vi "Data_get_joe_1.vi"() -> ()   [LabVIEW 2011]
uses:
  <vilib>/Analysis/2dsp.llb/Real FFT.vi
  <vilib>/Analysis/NI_AALPro.lvlib
panel:
  in  "Automatic Overwrite?":bool
  out "f cur. (GHz)":i32
  in  "TDS VISA Port":refnum<visa-resource-name>="GPIB0::1::INSTR"
  in  "Chirp up to (GHz)":dbl
  in  "PauseB":bool caption="Pause"
  in  "Substr":bool
  out "tdsavges#":i32 caption="tds averaged:"
  in  "Auto":bool caption="Autosave"
  in  "FFT every#":u32=1 min=1 max=1000 step=1
  in  "#steps":u32=1 min=1 step=1
  in  "f step (MHz)":dbl=0.0003 min=0.00025 max=67.0 step=1e-06 format="%#.12f"
  in  "time/point":T1(ring)
  in  "time/div":T2(ring)
  out "Current sweep":u32=1 min=1 max=1000 step=1
  in  "Ext":string="ccd"
  in  "Name":string="trace"
  in  "Folder":path
  in  "#Sweeps":u32=1 min=1 max=1000 step=1
  in  "Ampl. (dBm)":dbl min=-135.0 max=30.0 step=0.5 format="%#_8g"
  in  "f start (GHz)":dbl=0.0003 min=0.00025 max=67.0 step=1e-06 format="%#.12f"
  in  "Start":bool
  in  "Quit":bool
  in  "E8257D VISA Port":refnum<visa-resource-name>="GPIB0::1::INSTR"
  out "read time (ms)":u32
  out "#points":u32
  out "Busy":bool
  in  "Repetition rate (Hz)":ext=2.5
  in  "Chirp start (MHz)":ext=2.5
  in  "Filter up to (MHz)":ext=2.5
  in  "Amount of averagings":u32=10 min=1 step=1
  out "Data":dbl[](array[numeric])
  out "Frequency Domain Signal":cluster{ext[], dbl[]}(graph)
  out "FFT (Im)":dbl[](array[numeric])
  out "FFT (Re)":dbl[](array[numeric])
  out "Final array":ext[][](array[numeric])
  out "size(s)":i32
  out "Oscilloscope Data":dbl[](array[numeric])
  in  "Channel Number":u16=1
  out "Oscilloscope graph":dbl[](graph)
  in  "Stop":bool
  # "Oscilloscope TDS6124C"
  # "File Storage"
  # "PSG E8257D"
  # "Control"
  # "Spectrum data"
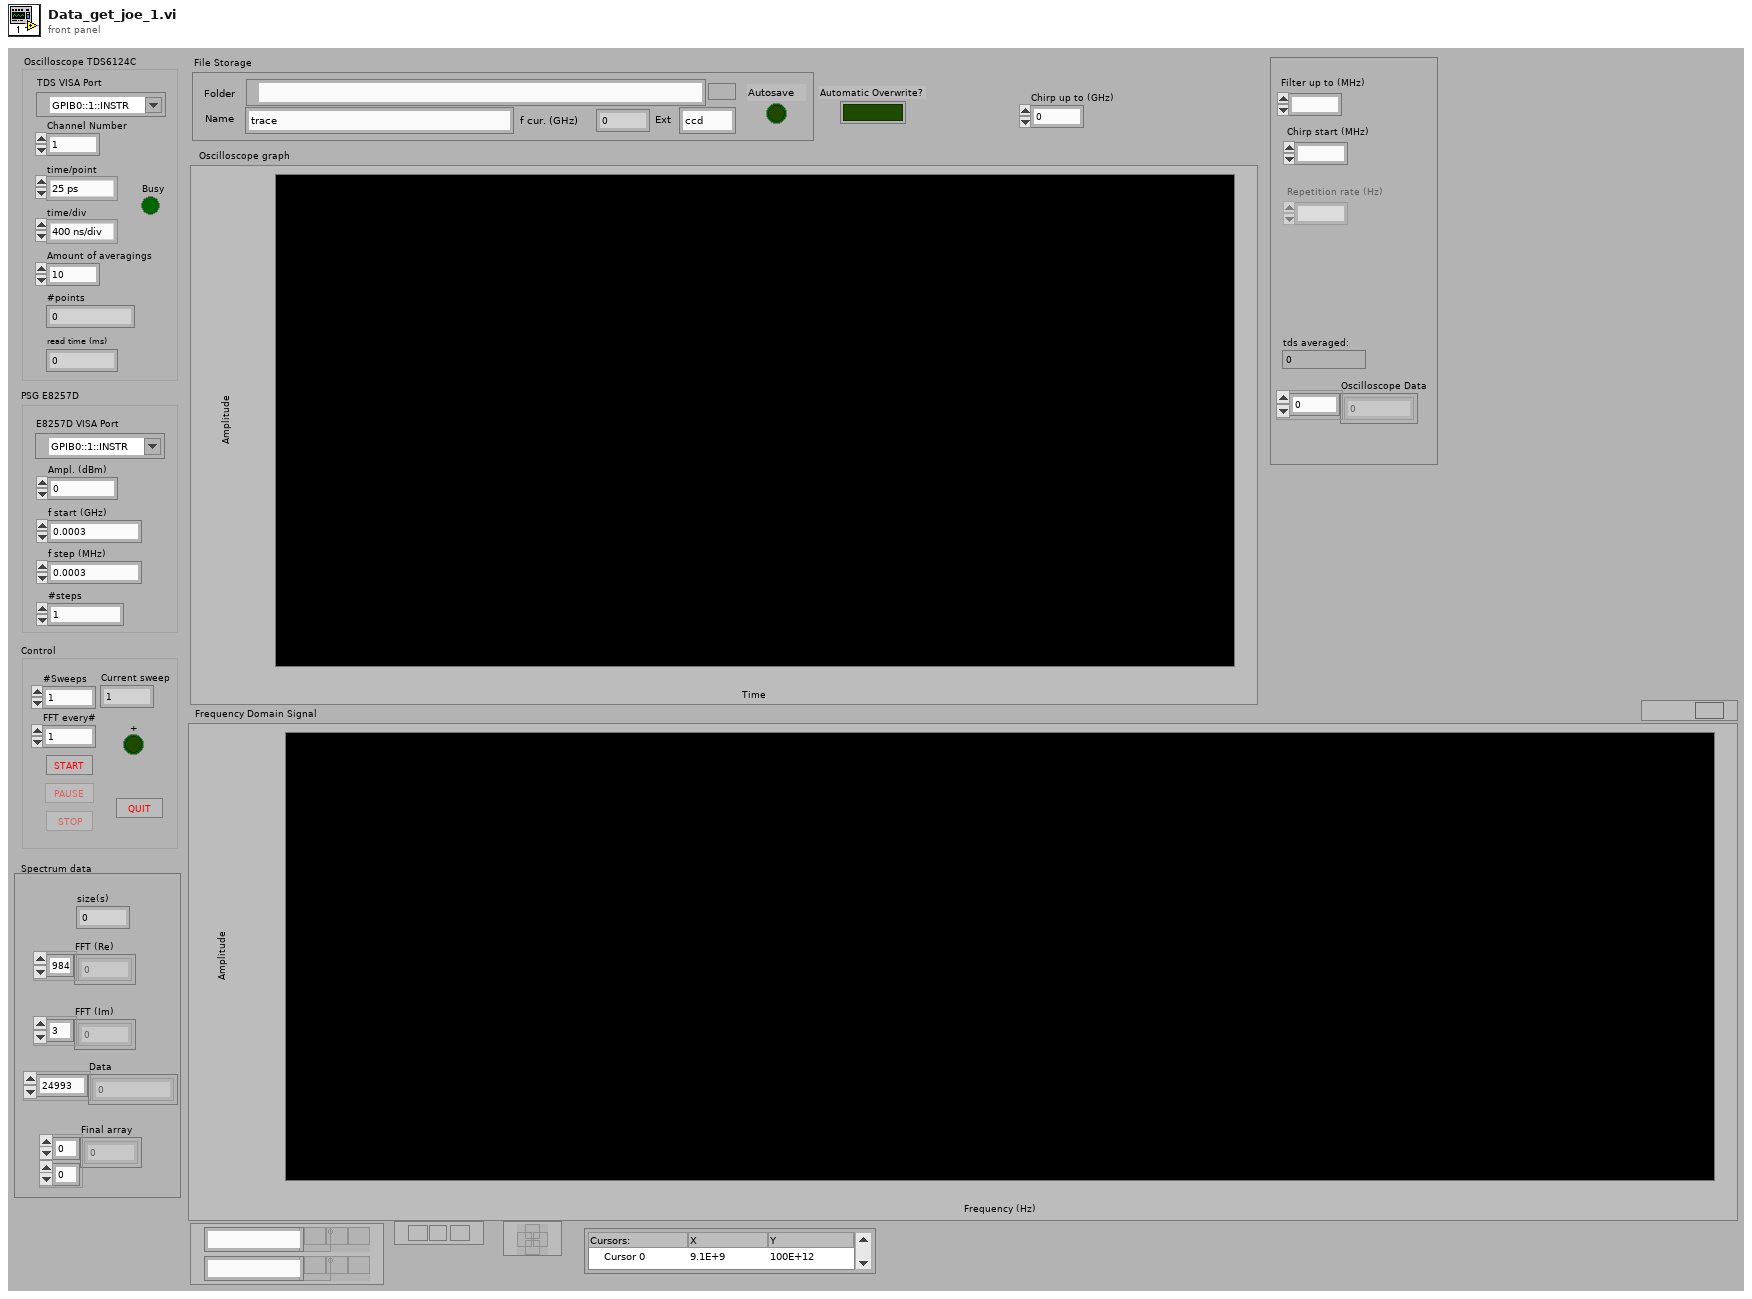
[diagram p1: front panel]
types:
  T1 = enum16{"25 ps", "50 ps", "100 ps", "200 ps", "400 ps", "800 ps", "2 ns"}
  T2 = enum16{"400 ns/div", "1 us/div", "2 us/div", "4 us/div", "10 us/div", "20 us/div"}
  T3 = enum8{"Enabled", "Disabled", "Disabled and Grayed Out"}
  T4 = enum16{"open", "replace", "create", "open or create", "replace or create", "replace or create with confirmation"}
  T5 = cluster{"Folder":path, "Name":string, "Ext":string}
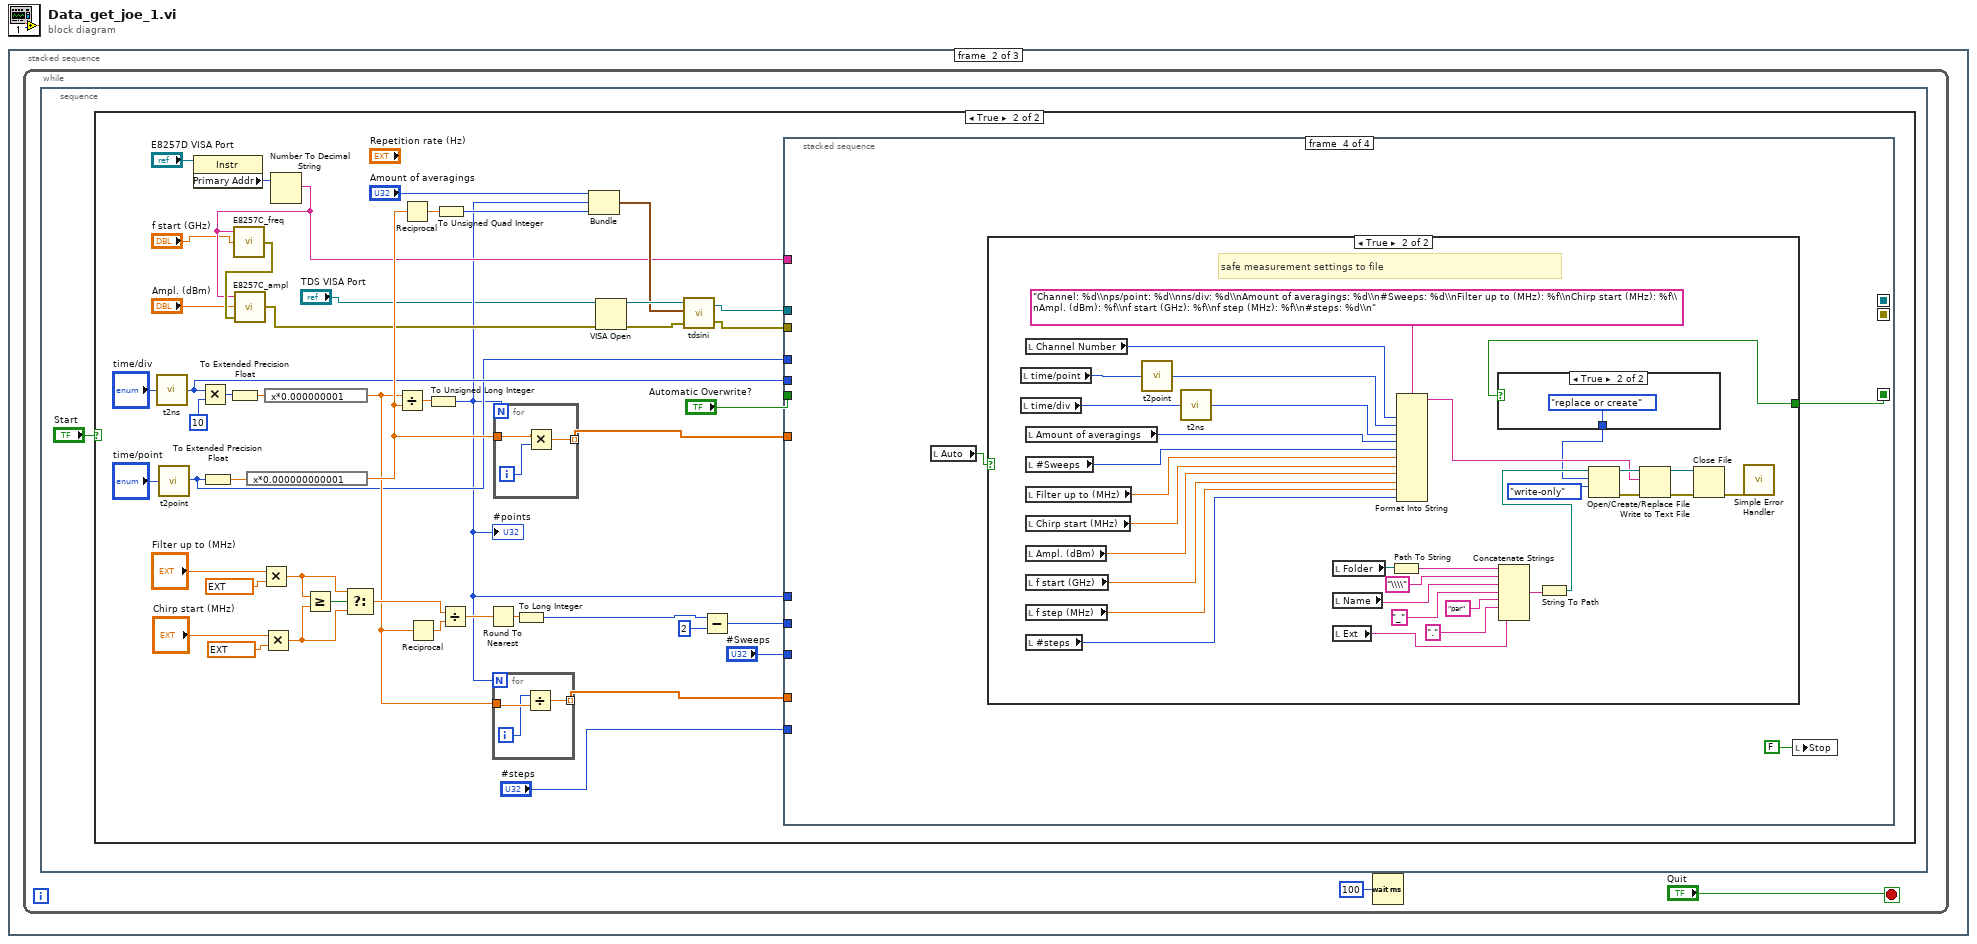
[diagram p0: block diagram]
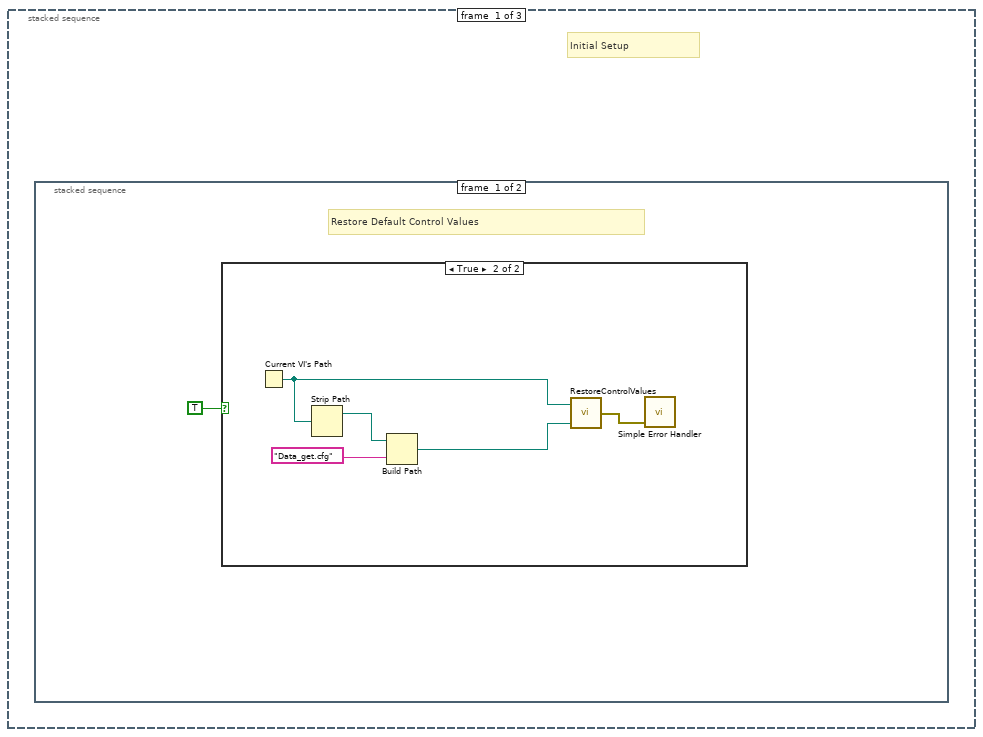
[diagram p2: hidden frame]
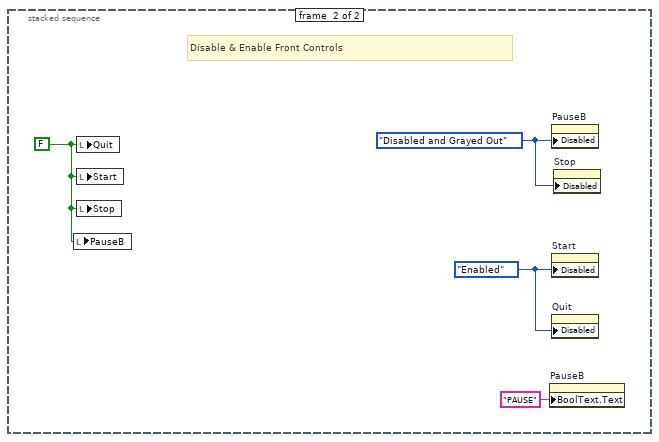
[diagram p4: hidden frame]
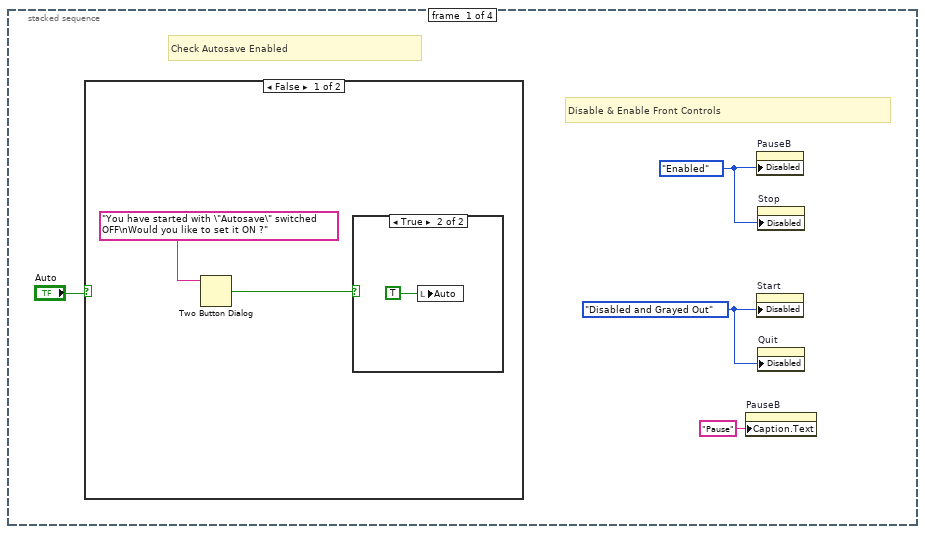
[diagram p6: hidden frame]
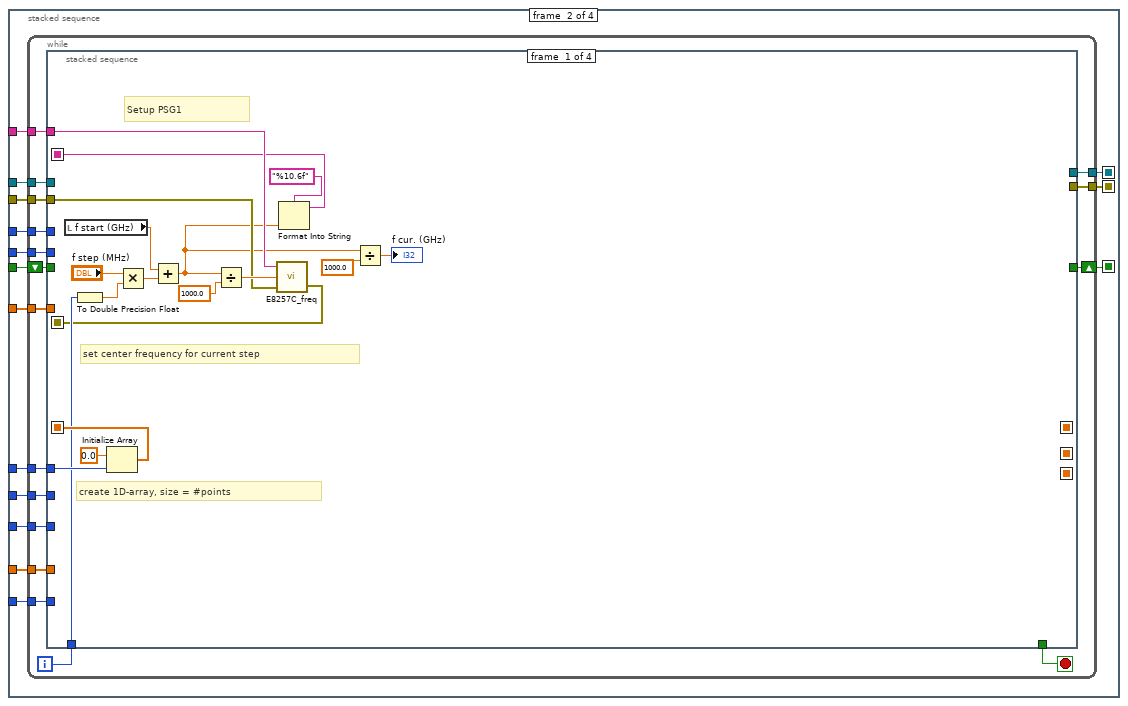
[diagram p9: hidden frame]
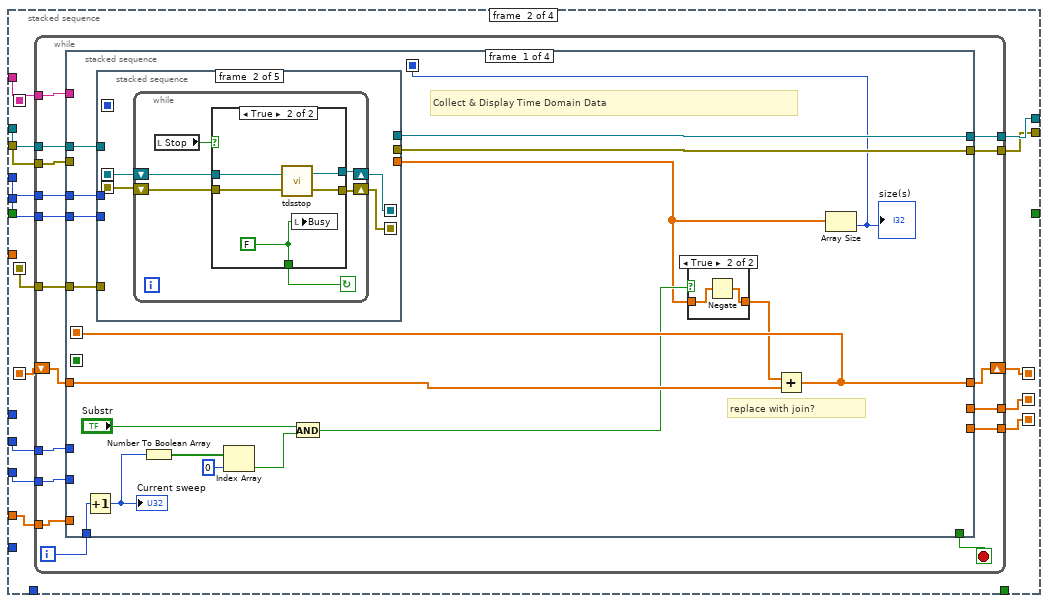
[diagram p10: hidden frame]
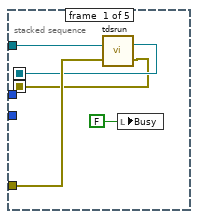
[diagram p12: hidden frame]
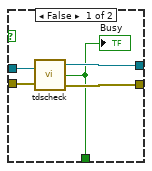
[diagram p13: hidden frame]
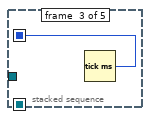
[diagram p14: hidden frame]
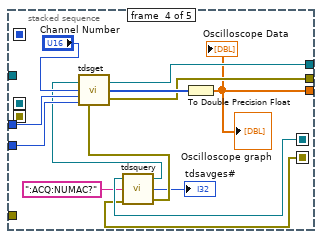
[diagram p15: hidden frame]
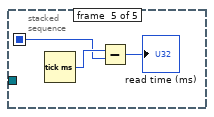
[diagram p16: hidden frame]
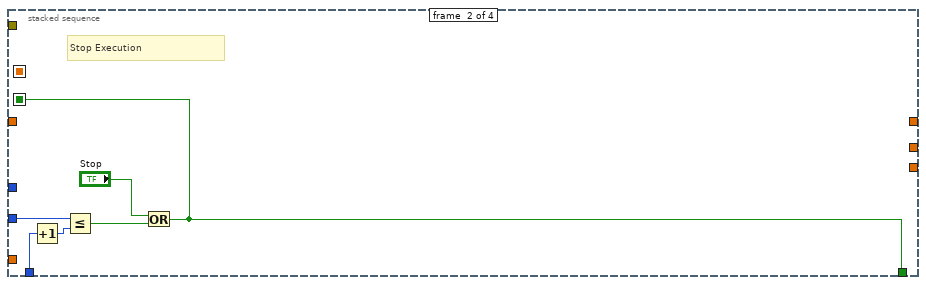
[diagram p17: hidden frame]
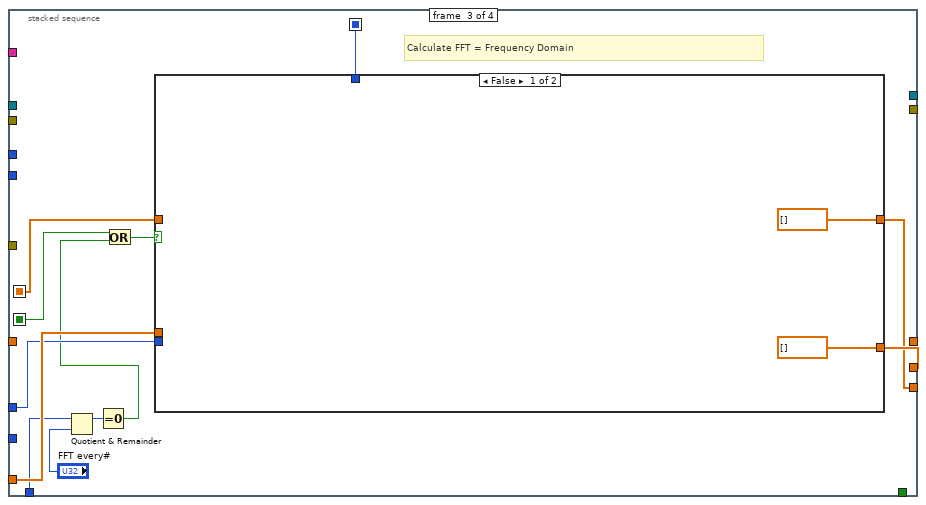
[diagram p18: hidden frame]
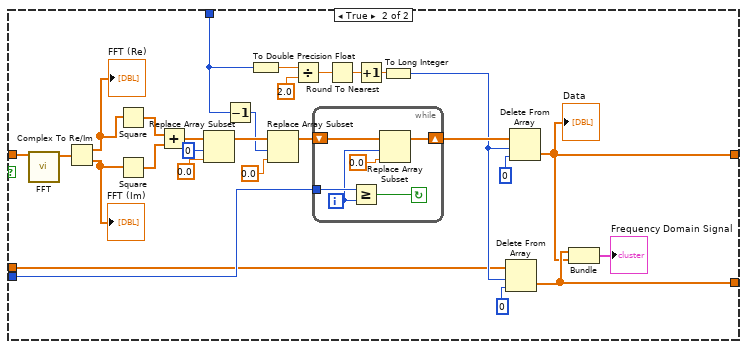
[diagram p19: hidden frame]
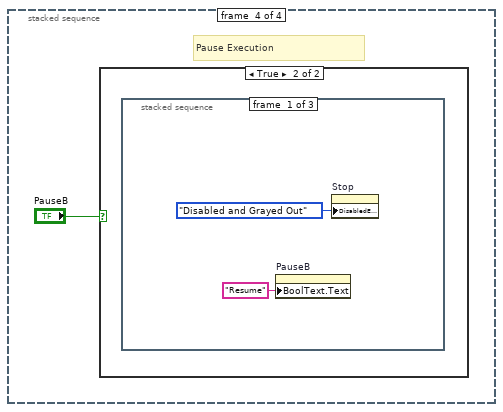
[diagram p20: hidden frame]
diagram:
  n1 = stacked-sequence {
    frame #0 {
      # "Initial Setup"
      n2 = stacked-sequence {
        frame #0 {
          # "Restore Default Control Values"
          n3 = case shown="True" TRUE {
            frame False {
            }
            frame True {
              n4 = Current VI's Path() -> (path=w2:path)
              n5 = Strip Path(path=w2) -> (stripped path=w3:path)  [unwired: 1 out]
              n6 = Build Path(base path=w3, name or relative path="Data_get.cfg") -> (appended path=w5:path)
              n7 = call "RestoreControlValues.vi"("file path"=w5, "vi path"=w2) -> ("error out"=w4:errorcluster)
              n8 = call <vilib>:"Simple Error Handler.vi"("error in (no error)"=w4) -> ()  [unwired: 4 in, 5 out]
            }
          }
        }
        frame #1 {
          w9 = T3."Disabled and Grayed Out" ("Disabled")
          w7 = T3."Enabled" ("Disabled")
          w10 = FALSE ("Quit")
          # "Disable & Enable Front Controls"
          n9 = local write "PauseB"(w10) -> ()
          n10 = local write "Quit"(w10) -> ()
          n11 = local write "Start"(w10) -> ()
          n12 = local write "Stop"(w10) -> ()
          n13 = property on="PauseB" class="Bool (strict)"("BoolText.Text"="PAUSE" ("Boolean Text.Text")) -> ()  [unwired: 2 in, 2 out]
          n14 = property on="PauseB" class="Bool (strict)"("Disabled"=w9) -> ()  [unwired: 2 in, 2 out]
          n15 = property on="Start" class="Bool (strict)"("Disabled"=w7) -> ()  [unwired: 2 in, 2 out]
          n16 = property on="Quit" class="Bool (strict)"("Disabled"=w7) -> ()  [unwired: 2 in, 2 out]
          n17 = property on="Stop" class="Bool (strict)"("Disabled"=w9) -> ()  [unwired: 2 in, 2 out]
        }
      }
    }
    frame #1 {
      n18 = while {
        stop <- "Quit" stop-if-true
        n19 = stacked-sequence {
          frame #0 {
            n20 = case shown="True" "Start" {
              frame False {
              }
              frame True {
                n21 = call "t2ns.vi"("t/div"="time/div") -> ("ns/div"=w26:u32)
                n22 = call "t2point.vi"("t/point"="time/point") -> ("ps/point"=w24:u32)
                n23 = property class="Instr"(reference="E8257D VISA Port") -> ("Primary Addr"=w32:u16)  [unwired: 1 in, 2 out]
                n24 = Multiply(x=w26, y=u32 10) -> (x*y=w55:u32)
                n25 = To Extended Precision Float(1:w24) -> (0:w52:ext)
                n26 = To Extended Precision Float(1:w55) -> (0:w53:ext)
                n27 = expression code="x*0.000000000001"(w52) -> (w38:ext)
                n28 = Multiply(x="Filter up to (MHz)", y=ext 1000000.0) -> (x*y=w44:ext)
                n29 = Multiply(x="Chirp start (MHz)", y=ext 1000000.0) -> (x*y=w41:ext)
                n30 = expression code="x*0.000000001"(w53) -> (w34:ext)
                n31 = Number To Decimal String(number=w32) -> (decimal integer string=w30:string)  [unwired: 1 in]
                n32 = call "E8257C_freq.vi"("Frequency GHz"="f start (GHz)", "GPIB address"=w30) -> ("error out"=w31:errorcluster)  [unwired: 1 in]
                n33 = call "E8257C_ampl.vi"("error in"=w31, "Amplitude dBm"="Ampl. (dBm)", "GPIB address"=w30) -> ("error out"=w29:errorcluster)
                n34 = Greater Or Equal?(x=w44, y=w41) -> (x >= y?=w51:bool)
                n35 = Select(t=w44, s=w51, f=w41) -> (s? t:f=w49:ext)
                n36 = Divide(x=w34, y=w38) -> (x/y=w54:ext)
                n37 = Reciprocal(x=w38) -> (1/x=w36:ext)
                n38 = Reciprocal(x=w34) -> (1/x=w50:ext)
                n39 = To Unsigned Long Integer(number=w54) -> (unsigned 32bit integer=w22:u32)
                "#points" <- w22
                n40 = To Unsigned Quad Integer(1:w36) -> (0:w37:u64)
                n41 = Divide(x=w49, y=w50) -> (x/y=w48:ext)
                n42 = Round To Nearest(number=w48) -> (nearest integer value=w47:ext)
                n43 = for {
                  N: w22 -> [_]
                  tunnel: w34 -> [w467]
                  tunnel: [w468] -> w35 mode=indexing
                  i -> [w466]
                  n44 = Divide(x=w466, y=w467) -> (x/y=w468:ext)
                }
                n45 = for {
                  N: w22 -> [_]
                  tunnel: w38 -> [w471]
                  tunnel: [w470] -> w27 mode=indexing
                  i -> [w469]
                  n46 = Multiply(x=w471, y=w469) -> (x*y=w470:ext)
                }
                n47 = To Long Integer(number=w47) -> (32bit integer=w19:i32)
                n48 = Bundle("Amount of averagings"="Amount of averagings", w22, w37) -> (w39:cluster{"Amount of averagings ":u32, u32, u64})  [unwired: 1 in]
                n49 = VISA Open(error in (no error)=w29, VISA resource name="TDS VISA Port") -> (VISA resource name=w57:refnum<visa-resource-name>, error out=w58:errorcluster)  [unwired: 3 in]
                n50 = call "tdsini.vi"("Error In (No Error)"=w58, "Acq_par"=w39, "VISA Port In"=w57) -> ("Error Out"=w59:errorcluster, "VISA Port Out"=w60:refnum<visa-resource-name>)
                n51 = Subtract(x=w19, y=2) -> (x-y=w17:i32)
                n52 = stacked-sequence {
                  seq-local: [_ w74 _ _] -> [_ _ w427 _]
                  seq-local: [_ w73 _ _] -> [_ _ w426 _]
                  seq-local: [_ w68 _ _] -> [_ _ _ w428]
                  tunnel: w60 -> [_ w82 _ _]
                  tunnel: w59 -> [_ w81 _ _]
                  tunnel: w24 -> [_ w80 _ _]
                  tunnel: w26 -> [_ w79 _ _]
                  tunnel: w17 -> [_ w78 _ _]
                  tunnel: w35 -> [_ w77 _ _]
                  tunnel: w30 -> [_ w76 w424 _]
                  tunnel: "#Sweeps" -> [_ w75 _ _]
                  tunnel: w27 -> [_ w70 _ _]
                  tunnel: w22 -> [_ w72 _ _]
                  tunnel: "#steps" -> [_ w71 _ _]
                  tunnel: "Automatic Overwrite?" -> [_ w69 _ _]
                  frame #0 {
                    w62 = T3."Enabled" ("Disabled")
                    w61 = T3."Disabled and Grayed Out" ("Disabled")
                    # "Check Autosave Enabled"
                    # "Disable & Enable Front Controls"
                    n53 = case shown="False" "Auto" {
                      frame False {
                        n54 = Two Button Dialog(message="You have started with \"Autosave\" switched OFF\nWould you like to set it ON ?") -> (T button?=w65:bool)  [unwired: 2 in]
                        n55 = case shown="True" w65 {
                          frame False {
                          }
                          frame True {
                            n56 = local write "Auto"(TRUE) -> ()
                          }
                        }
                      }
                      frame True {
                      }
                    }
                    n57 = property on="PauseB" class="Bool (strict)"("Caption.Text"="Pause") -> ()  [unwired: 2 in, 2 out]
                    n58 = property on="PauseB" class="Bool (strict)"("Disabled"=w62) -> ()  [unwired: 2 in, 2 out]
                    n59 = property on="Start" class="Bool (strict)"("Disabled"=w61) -> ()  [unwired: 2 in, 2 out]
                    n60 = property on="Stop" class="Bool (strict)"("Disabled"=w62) -> ()  [unwired: 2 in, 2 out]
                    n61 = property on="Quit" class="Bool (strict)"("Disabled"=w61) -> ()  [unwired: 2 in, 2 out]
                  }
                  frame #1 {
                    n62 = while {
                      tunnel: w82 -> [w99]
                      tunnel: w81 -> [w98]
                      tunnel: w80 -> [w97]
                      tunnel: w79 -> [w96]
                      tunnel: w78 -> [w95]
                      tunnel: w77 -> [w94]
                      tunnel: w76 -> [w93]
                      tunnel: w75 -> [w92]
                      tunnel: [w91] -> w74
                      tunnel: [w90] -> w73
                      tunnel: w72 -> [w89]
                      tunnel: w71 -> [w87]
                      tunnel: w70 -> [w85]
                      shift-right: [w83] -> w68
                      shift-left: w69 -> [w84]
                      i -> [w88]
                      stop <- w86 stop-if-true
                      n63 = stacked-sequence {
                        seq-local: [w116 _ _ _] -> [_ w122 _ _]
                        seq-local: [w105 _ _ _] -> [_ w121 _ _]
                        seq-local: [_ w120 _ _] -> [_ _ w280 _]
                        seq-local: [_ w119 _ _] -> [_ _ w279 _]
                        seq-local: [_ w118 _ _] -> [_ _ w278 _]
                        seq-local: [w103 _ _ _] -> [_ _ w277 _]
                        tunnel: w99 -> [_ w132 _ _]
                        tunnel: w98 -> [w106 w131 _ _]
                        tunnel: w97 -> [_ w130 _ _]
                        tunnel: w96 -> [_ w129 _ _]
                        tunnel: w95 -> [_ w128 _ _]
                        tunnel: w94 -> [_ w127 _ _]
                        tunnel: w93 -> [w107 w126 _ _]
                        tunnel: w92 -> [_ w125 _ _]
                        tunnel: [_ w124 _ _] -> w91
                        tunnel: [_ w123 _ _] -> w90
                        tunnel: w89 -> [w115 _ _ _]
                        tunnel: w88 -> [w110 _ _ w418]
                        tunnel: w87 -> [_ _ _ w417]
                        tunnel: [_ _ _ w416] -> w86
                        tunnel: w85 -> [_ _ w281 _]
                        tunnel: w84 -> [_ _ w275 _]
                        tunnel: [_ _ w274 _] -> w83
                        frame #0 {
                          # "Setup PSG1"
                          # "create 1D-array, size = #points"
                          # "set center frequency for current step"
                          n64 = local read "f start (GHz)"() -> (w108:dbl)
                          n65 = To Double Precision Float(number=w110) -> (double precision float=w111:dbl)
                          n66 = Initialize Array(0.0 ("element"), w115) -> (w116:dbl[])
                          n67 = Multiply(x="f step (MHz)", y=w111) -> (x*y=w109:dbl)
                          n68 = Add(x=w108, y=w109) -> (x+y=w101:dbl)
                          n69 = Divide(x=w101, y=1000.0) -> (x/y=w114:dbl)
                          n70 = call "E8257C_freq.vi"("error in"=w106, "Frequency GHz"=w114, "GPIB address"=w107) -> ("error out"=w105:errorcluster)
                          n71 = Format Into String(format string="%10.6f", w101) -> (resulting string=w103:string)  [unwired: 2 in, 1 out]
                          n72 = Divide(x=w101, y=1000.0) -> (x/y=→"f cur. (GHz)":dbl)
                        }
                        frame #1 {
                          n73 = while {
                            tunnel: [w146] -> w123
                            tunnel: [w147] -> w124
                            tunnel: w131 -> [w148]
                            tunnel: w132 -> [w149]
                            tunnel: w130 -> [w145]
                            tunnel: w129 -> [w144]
                            tunnel: w127 -> [w142]
                            tunnel: w128 -> [w143]
                            tunnel: w126 -> [w139]
                            tunnel: w125 -> [w138]
                            shift-right: [w136] -> w120
                            shift-left: w122 -> [w137]
                            tunnel: [w135] -> w119
                            tunnel: w121 -> [w134]
                            tunnel: [w133] -> w118
                            i -> [w141]
                            stop <- w140 stop-if-true
                            n74 = stacked-sequence {
                              seq-local: [w159 _ _ _] -> [_ _ w230 _]
                              seq-local: [w160 _ _ _] -> [_ _ w229 _]
                              seq-local: [_ w213 _ _] -> [_ _ w220 _]
                              tunnel: w149 -> [w167 _ _ _]
                              tunnel: w148 -> [_ _ _ _]
                              tunnel: [w166 _ _ _] -> w147
                              tunnel: [w165 _ _ _] -> w146
                              tunnel: w145 -> [w164 _ _ _]
                              tunnel: w144 -> [w163 _ _ _]
                              tunnel: w143 -> [_ _ w227 _]
                              tunnel: w142 -> [_ _ w228 _]
                              tunnel: w141 -> [w158 w218 w224 _]
                              tunnel: [_ w213 _ _] -> w140
                              tunnel: w139 -> [_ _ _ _]
                              tunnel: w138 -> [_ w215 _ _]
                              tunnel: w137 -> [w162 _ _ _]
                              tunnel: [w160 _ _ _] -> w136
                              tunnel: [_ _ w226 _] -> w135
                              tunnel: w134 -> [w161 _ _ _]
                              tunnel: [_ _ w225 _] -> w133
                              frame #0 {
                                # "replace with join?"
                                # "Collect & Display Time Domain Data"
                                n75 = Increment(x=w158) -> (x+1=w150:i32)
                                "Current sweep" <- w150
                                n76 = stacked-sequence {
                                seq-local: [w173 _ _ _ _] -> [_ w179 _ _ _]
                                seq-local: [w172 _ _ _ _] -> [_ w178 _ _ _]
                                seq-local: [_ w176 _ _ _] -> [_ _ _ w201 _]
                                seq-local: [_ w177 _ _ _] -> [_ _ _ w202 _]
                                seq-local: [_ _ w196 _ _] -> [_ _ _ _ w211]
                                tunnel: w167 -> [w174 _ _ _ _]
                                tunnel: w161 -> [w175 _ _ _ _]
                                tunnel: [_ _ _ w208 _] -> w166
                                tunnel: [_ _ _ w207 _] -> w165
                                tunnel: w164 -> [_ _ _ w205 _]
                                tunnel: w163 -> [_ _ _ w204 _]
                                tunnel: [_ _ _ w203 _] -> w153
                                frame #0 {
                                n77 = call "tdsrun.vi"("Error In (No Error)"=w175, "VISA Port In"=w174) -> ("Error Out"=w172:errorcluster, "VISA Port Out"=w173:refnum<visa-resource-name>)
                                n78 = local write "Busy"(FALSE ("Busy")) -> ()
                                }
                                frame #1 {
                                n79 = while {
                                shift-right: [w183] -> w177
                                shift-left: w179 -> [w184]
                                shift-right: [w182] -> w176
                                shift-left: w178 -> [w185]
                                stop <- w181 continue-if-true
                                n80 = local read "Stop"() -> (w180:bool)
                                n81 = case shown="True" w180 {
                                tunnel: w185 -> [w190 w194]
                                tunnel: w184 -> [w189 w195]
                                tunnel: [w188 w192] -> w183
                                tunnel: [w187 w193] -> w182
                                tunnel: [w186 w191] -> w181
                                frame False {
                                n82 = call "tdscheck.vi"("VISA Port In"=w189, "Error In (No Error)"=w190) -> ("VISA Port Out"=w188:refnum<visa-resource-name>, "busy"=w186:bool, "Error Out"=w187:errorcluster)
                                "Busy" <- w186
                                }
                                frame True {
                                w191 = FALSE ("busy")
                                n83 = call "tdsstop.vi"("Error In (No Error)"=w194, "VISA Port In"=w195) -> ("Error Out"=w193:errorcluster, "VISA Port Out"=w192:refnum<visa-resource-name>)
                                n84 = local write "Busy"(w191) -> ()
                                }
                                }
                                }
                                }
                                frame #2 {
                                n85 = Tick Count (ms)() -> (millisecond timer value=w196:u32)
                                }
                                frame #3 {
                                n86 = call "tdsquery.vi"("Error In (No Error)"=w201, "String to TDS"=":ACQ:NUMAC?", "VISA Port In"=w202) -> ("Error Out"=w198:errorcluster, "number"=→"tdsavges#":i32, "VISA Port Out"=w199:refnum<visa-resource-name>)
                                n87 = call "tdsget.vi"("VISA Port In"=w199, "Channel Number"="Channel Number", "ps/point"=w205, "ns/div"=w204, "Error In (No Error)"=w198) -> ("VISA Port Out"=w208:refnum<visa-resource-name>, "TDS Data"=w209:u16[], "Error Out"=w207:errorcluster)  [unwired: 8 in]
                                n88 = To Double Precision Float(number=w209) -> (double precision float=w203:dbl[])
                                "Oscilloscope graph" <- w203
                                "Oscilloscope Data" <- w203
                                }
                                frame #4 {
                                n89 = Tick Count (ms)() -> (millisecond timer value=w212:u32)
                                n90 = Subtract(x=w212, y=w211) -> (x-y=→"read time (ms)":u32)
                                }
                                }
                                n91 = Number To Boolean Array(number=w150) -> (Boolean array=w157:bool[])
                                n92 = Index Array(array=w157, index=0) -> (element=w155:bool)
                                n93 = And(x="Substr", y=w155) -> (x .and. y?=w154:bool)
                                n94 = case shown="True" w154 {
                                tunnel: w153 -> [w168 w170]
                                tunnel: [w168 w169] -> w152
                                frame False {
                                }
                                frame True {
                                n95 = Negate(x=w170) -> (-x=w169:dbl[])
                                }
                                }
                                n96 = Add(x=w152, y=w162) -> (x+y=w160:dbl[])
                                n97 = Array Size(array=w153) -> (size(s)=w159:i32)
                                "size(s)" <- w159
                              }
                              frame #1 {
                                # "Stop Execution"
                                n98 = Increment(x=w218) -> (x+1=w214:i32)
                                n99 = Less Or Equal?(x=w215, y=w214) -> (x <= y?=w217:bool)
                                n100 = Or(x="Stop", y=w217) -> (x .or. y?=w213:bool)
                              }
                              frame #2 {
                                # "Calculate FFT = Frequency Domain"
                                n101 = Quotient & Remainder(x=w224, y="FFT every#") -> (x-y*floor(x/y)=w222:u32)  [unwired: 1 out]
                                n102 = Equal To 0?(x=w222) -> (x = 0?=w219:bool)
                                n103 = Or(x=w220, y=w219) -> (x .or. y?=w221:bool)
                                n104 = case shown="False" w221 {
                                tunnel: w230 -> [_ w238]
                                tunnel: w229 -> [_ w237]
                                tunnel: w228 -> [_ w233]
                                tunnel: w227 -> [_ w236]
                                tunnel: [ext[] [] w235] -> w226
                                tunnel: [dbl[] [] w234] -> w225
                                frame False {
                                }
                                frame True {
                                n105 = call-poly <vilib>:"FFT.vi"("X"=w237) -> ("FFT {X}"=w260:cdb[])  [unwired: 9 in, 1 out]
                                n106 = Complex To Re/Im(x + iy=w260) -> (x=w259:dbl[], y=w258:dbl[])
                                "FFT (Re)" <- w259
                                "FFT (Im)" <- w258
                                n107 = Square(x=w259) -> (x^2=w257:dbl[])
                                n108 = Square(x=w258) -> (x^2=w256:dbl[])
                                n109 = Add(x=w257, y=w256) -> (x+y=w252:dbl[])
                                n110 = Replace Array Subset(array=w252, new element=0.0 ("new element/subarray"), index=0) -> (w251:dbl[])
                                n111 = Decrement(x=w238) -> (x-1=w250:i32)
                                n112 = To Double Precision Float(number=w238) -> (double precision float=w246:dbl)
                                n113 = Replace Array Subset(array=w251, new element=0.0 ("new element/subarray"), index=w250) -> (w248:dbl[])
                                n114 = Divide(x=w246, y=2.0) -> (x/y=w244:dbl)
                                n115 = while {
                                tunnel: w236 -> [w265]
                                shift-right: [w263] -> w247
                                shift-left: w248 -> [w264]
                                i -> [w262]
                                stop <- w266 continue-if-true
                                n116 = Greater Or Equal?(x=w265, y=w262) -> (x >= y?=w266:bool)
                                n117 = Replace Array Subset(array=w264, new element=0.0 ("new element/subarray"), index=w262) -> (w263:dbl[])
                                }
                                n118 = Round To Nearest(number=w244) -> (nearest integer value=w243:dbl)
                                n119 = Increment(x=w243) -> (x+1=w242:dbl)
                                n120 = To Long Integer(number=w242) -> (32bit integer=w239:i32)
                                n121 = Delete From Array(array=w233, length=w239, index=0) -> (deleted portion=w235:ext[])  [unwired: 1 out]
                                n122 = Delete From Array(array=w247, length=w239, index=0) -> (deleted portion=w234:dbl[])  [unwired: 1 out]
                                "Data" <- w234
                                n123 = Bundle(w235, w234) -> (→"Frequency Domain Signal":cluster{ext[], dbl[]})  [unwired: 1 in]
                                }
                                }
                              }
                              frame #3 {
                                # "Pause Execution"
                                n124 = case shown="True" "PauseB" {
                                frame False {
                                }
                                frame True {
                                n125 = stacked-sequence {
                                frame #0 {
                                n126 = property on="PauseB" class="Bool (strict)"("BoolText.Text"="Resume" ("Caption.Text")) -> ()  [unwired: 2 in, 2 out]
                                n127 = property on="Stop" class="Bool (strict)"("DisabledEnum"=T3."Disabled and Grayed Out" ("Disabled")) -> ()  [unwired: 2 in, 2 out]
                                }
                                frame #1 {
                                n128 = while {
                                stop <- w271 continue-if-true
                                n129 = local read "PauseB"() -> (w271:bool)
                                n130 = Wait Until Next ms Multiple(millisecond multiple=u32 150) -> ()  [unwired: 1 out]
                                }
                                }
                                frame #2 {
                                n131 = property on="PauseB" class="Bool (strict)"("BoolText.Text"="Pause" ("Caption.Text")) -> ()  [unwired: 2 in, 2 out]
                                n132 = property on="Stop" class="Bool (strict)"("DisabledEnum"=T3."Enabled" ("Disabled")) -> ()  [unwired: 2 in, 2 out]
                                }
                                }
                                }
                                }
                              }
                            }
                          }
                        }
                        frame #2 {
                          # "Auto Safe?"
                          n133 = local read "Auto"() -> (w276:bool)
                          n134 = case shown="True" w276 {
                            tunnel: w281 -> [_ w289]
                            tunnel: w280 -> [_ w288]
                            tunnel: w279 -> [_ w287]
                            tunnel: w278 -> [_ w286]
                            tunnel: w277 -> [_ w285]
                            tunnel: w275 -> [_ w284]
                            tunnel: [FALSE w283] -> w274
                            frame False {
                            }
                            frame True {
                              n135 = stacked-sequence {
                                seq-local: [w290 _ _ _] -> [_ w314 _ _]
                                seq-local: [_ _ w368 _] -> [_ _ _ w408]
                                seq-local: [_ w300 _ _] -> [_ _ _ w399]
                                tunnel: w289 -> [_ w316 _ _]
                                tunnel: w288 -> [_ w303 _ _]
                                tunnel: w287 -> [_ _ _ w411]
                                tunnel: w286 -> [_ _ _ w410]
                                tunnel: w285 -> [w293 w302 w370 _]
                                tunnel: w284 -> [_ w306 _ _]
                                tunnel: [_ w300 _ _] -> w283
                                frame #0 {
                                # "create complete filename incl. path as a string"
                                n136 = Path To String(path="Folder") -> (string=w298:string)
                                n137 = Concatenate Strings(w298, "\\\\" ("string"), "Name", "_", "td", w293, ".", "Ext") -> (w290:string)
                                }
                                frame #1 {
                                # "(%e) = Scientific Notation"
                                n138 = Build Array(w316, w303) -> (w318:ext[][])
                                n139 = String To Path(string=w314) -> (path=w305:path)
                                n140 = case shown="False" w306 {
                                tunnel: w314 -> [w320 _]
                                tunnel: [w325 w366] -> w300
                                tunnel: [w323 T4."replace or create" ("operation (0:open)")] -> w308
                                tunnel: w306 -> [w324 w366]
                                tunnel: w305 -> [w322 w365]
                                tunnel: [w321 w365] -> w304
                                tunnel: w302 -> [w319 _]
                                frame False {
                                n141 = call "CheckFileExist.vi"("Path"=w320) -> ("File Exists"=w327:bool, "Overwrite File"=w326:bool)  [unwired: 1 in, 1 out]
                                n142 = case "check file existance" shown="True" w327 {
                                tunnel: w326 -> [_ w336]
                                tunnel: [w330 w334] -> w325
                                tunnel: w324 -> [w330 _]
                                tunnel: [T4."create" ("operation (0:open)") w335] -> w323
                                tunnel: w322 -> [w328 w333]
                                tunnel: [w328 w332] -> w321
                                tunnel: w319 -> [_ w331]
                                frame False {
                                # "file doesn't exist"
                                }
                                frame True {
                                # "file exists"
                                n143 = case shown="False" w336 {
                                tunnel: [w339 T4."replace or create" ("operation (0:open)")] -> w335
                                tunnel: [w340 TRUE] -> w334
                                tunnel: w333 -> [_ w362]
                                tunnel: [w337 w362] -> w332
                                tunnel: w331 -> [w338 _]
                                frame False {
                                # "file exists and should not be overwritten"
                                n144 = stacked-sequence {
                                tunnel: [_ _ FALSE] -> w340
                                tunnel: [_ _ T4."create" ("operation (0:open)")] -> w339
                                tunnel: w338 -> [_ w349 _]
                                tunnel: [_ w354 _] -> w337
                                frame #0 {
                                # "enter new file name"
                                n145 = local read "Folder"() -> (w348:path)
                                n146 = local read "Name"() -> (w347:string)
                                n147 = local read "Ext"() -> (w346:string)
                                n148 = Bundle("Folder"=w348, "Name"=w347, "Ext"=w346) -> (w345:T5)  [unwired: 1 in]
                                n149 = call "ChangeFileName.vi"("input par"=w345) -> ("output par"=w344:T5)  [unwired: 1 out]
                                n150 = Unbundle(w344) -> ("Folder"=w343:path, "Name"=w342:string, "Ext"=w341:string)
                                n151 = local write "Folder"(w343) -> ()
                                n152 = local write "Name"(w342) -> ()
                                n153 = local write "Ext"(w341) -> ()
                                }
                                frame #1 {
                                # "create new path"
                                n154 = local read "Ext"() -> (w351:string)
                                n155 = local read "Folder"() -> (w356:path)
                                n156 = local read "Name"() -> (w355:string)
                                n157 = Path To String(path=w356) -> (string=w359:string)
                                n158 = Concatenate Strings(w359, "\\\\" ("string"), w355, "_", "td", w349, ".", w351) -> (w350:string)
                                n159 = String To Path(string=w350) -> (path=w354:path)
                                }
                                frame #2 {
                                }
                                }
                                }
                                frame True {
                                # "overwrite existing file"
                                }
                                }
                                }
                                }
                                }
                                frame True {
                                }
                                }
                                n160 = Transpose 2D Array(2D array=w318) -> (transposed array=w315:ext[][])
                                n161 = Array To Spreadsheet String(array=w315, 3:"%e") -> (spreadsheet string=w307:string)  [unwired: 1 in]
                                n162 = Open/Create/Replace File(file path (use dialog)=w304, operation (0:open)=w308, access (0:read/write)=enum16{"read/write", "read-only", "write-only"}."write-only") -> (refnum out=w310:refnum<file>, error out=w313:errorcluster)  [unwired: 3 in, 1 out]
                                n163 = Write to Text File(file (use dialog)=w310, text=w307, error in=w313) -> (refnum out=w311:refnum<file>, error out=w312:errorcluster)  [unwired: 1 in, 1 out]
                                n164 = Close File(refnum=w311, error in=w312) -> (error out=w301:errorcluster)  [unwired: 1 out]
                                n165 = call <vilib>:"Simple Error Handler.vi"("error in (no error)"=w301) -> ()  [unwired: 4 in, 5 out]
                                }
                                frame #2 {
                                n166 = local read "Folder"() -> (w372:path)
                                n167 = local read "Name"() -> (w371:string)
                                n168 = local read "Ext"() -> (w369:string)
                                n169 = Path To String(path=w372) -> (string=w378:string)
                                n170 = Concatenate Strings(w378, "\\\\" ("string"), w371, "_") -> (w373:string)
                                n171 = Concatenate Strings(w373, "sd", w370, ".", w369) -> (w368:string)
                                }
                                frame #3 {
                                n172 = Multiply(x="Chirp up to (GHz)", y=1000000000.0) -> (x*y=w380:dbl)
                                n173 = To Extended Precision Float(1:w380) -> (0:w379:ext)
                                n174 = To Extended Precision Float(1:w410) -> (0:w412:ext[])
                                n175 = Build Array(w411, w412) -> (w409:ext[][])
                                n176 = String To Path(string=w408) -> (path=w401:path)
                                n177 = case shown="True" w399 {
                                tunnel: [T4."replace or create with confirmation" ("operation (0:open)") T4."replace or create" ("operation (0:open)")] -> w400
                                frame False {
                                }
                                frame True {
                                }
                                }
                                n178 = Transpose 2D Array(2D array=w409) -> (transposed array=w382:ext[][])
                                n179 = Index Array(array=w382, index (col)=0 ("disabled index (col)")) -> (element=w392:ext[])  [unwired: 1 in]
                                n180 = Index Array(array=w392, index=1) -> (element=w394:ext)
                                n181 = Index Array(array=w392, index=0) -> (element=w393:ext)
                                n182 = Subtract(x=w394, y=w393) -> (x-y=w389:ext)
                                n183 = Divide(x=w379, y=w389) -> (x/y=w386:ext)
                                n184 = Round To Nearest(number=w386) -> (nearest integer value=w388:ext)
                                n185 = To Long Integer(number=w388) -> (32bit integer=w387:i32)
                                n186 = Increment(x=w387) -> (x+1=w383:i32)
                                n187 = Array Subset(array=w382, index (row)=0 ("index"), length (row)=w383, index (col)=0 ("index"), length (col)=w383) -> (w381:ext[][])
                                "Final array" <- w381
                                n188 = Array To Spreadsheet String(array=w381, 3:"%e") -> (spreadsheet string=w402:string)  [unwired: 1 in]
                                n189 = Open/Create/Replace File(file path (use dialog)=w401, operation (0:open)=w400, access (0:read/write)=enum16{"read/write", "read-only", "write-only"}."write-only") -> (refnum out=w404:refnum<file>, error out=w407:errorcluster)  [unwired: 3 in, 1 out]
                                n190 = Write to Text File(file (use dialog)=w404, text=w402, error in=w407) -> (refnum out=w405:refnum<file>, error out=w406:errorcluster)  [unwired: 1 in, 1 out]
                                n191 = Close File(refnum=w405, error in=w406) -> (error out=w398:errorcluster)  [unwired: 1 out]
                                n192 = call <vilib>:"Simple Error Handler.vi"("error in (no error)"=w398) -> ()  [unwired: 4 in, 5 out]
                                }
                              }
                            }
                          }
                        }
                        frame #3 {
                          n193 = Increment(x=w418) -> (x+1=w420:i32)
                          n194 = Less Or Equal?(x=w417, y=w420) -> (x <= y?=w421:bool)
                          n195 = local read "Stop"() -> (w419:bool)
                          n196 = Or(x=w419, y=w421) -> (x .or. y?=w416:bool)
                        }
                      }
                    }
                  }
                  frame #2 {
                    w423 = T3."Disabled and Grayed Out" ("Disabled")
                    w422 = T3."Enabled" ("Disabled")
                    n197 = call "E8257C_local.vi"("GPIB address"=w424) -> ("error out"=w425:errorcluster)  [unwired: 1 in]
                    n198 = call <vilib>:"Simple Error Handler.vi"("error in (no error)"=w425) -> ()  [unwired: 4 in, 5 out]
                    n199 = property on="Quit" class="Bool (strict)"("Disabled"=w422) -> ()  [unwired: 2 in, 2 out]
                    n200 = property on="PauseB" class="Bool (strict)"("Disabled"=w423) -> ()  [unwired: 2 in, 2 out]
                    n201 = property on="Stop" class="Bool (strict)"("Disabled"=w423) -> ()  [unwired: 2 in, 2 out]
                    n202 = property on="Start" class="Bool (strict)"("Disabled"=w422) -> ()  [unwired: 2 in, 2 out]
                    n203 = VISA Close(VISA resource name=w427, error in (no error)=w426) -> ()  [unwired: 1 out]
                  }
                  frame #3 {
                    n204 = local read "Auto"() -> (w429:bool)
                    n205 = case shown="True" w429 {
                      tunnel: w428 -> [_ w432]
                      frame False {
                      }
                      frame True {
                        # "safe measurement settings to file"
                        n206 = local read "time/point"() -> (w461:T1)
                        n207 = local read "time/div"() -> (w460:T2)
                        n208 = local read "Channel Number"() -> (w462:u16)
                        n209 = local read "Amount of averagings"() -> (w459:u32)
                        n210 = local read "#Sweeps"() -> (w458:u32)
                        n211 = local read "Filter up to (MHz)"() -> (w457:ext)
                        n212 = local read "Chirp start (MHz)"() -> (w456:ext)
                        n213 = local read "Ampl. (dBm)"() -> (w455:dbl)
                        n214 = local read "f start (GHz)"() -> (w452:dbl)
                        n215 = local read "f step (MHz)"() -> (w451:dbl)
                        n216 = local read "#steps"() -> (w450:u32)
                        n217 = call "t2point.vi"("t/point"=w461) -> ("ps/point"=w453:u32)
                        n218 = call "t2ns.vi"("t/div"=w460) -> ("ns/div"=w454:u32)
                        n219 = local read "Folder"() -> (w446:path)
                        n220 = local read "Name"() -> (w445:string)
                        n221 = local read "Ext"() -> (w442:string)
                        n222 = Path To String(path=w446) -> (string=w449:string)
                        n223 = Format Into String(format string="Channel: %d\\nps/point: %d\\nns/div: %d\\nAmount of averagings: %d\\n#Sweeps: %d\\nFilter up to (MHz): %f\\nChirp start (MHz): %f\\nAmpl. (dBm): %f\\nf start (GHz): %f\\nf step (MHz): %f\\n#steps: %d\\n", w462, w453, w454, w459, w458, w457, w456, w455, w452, w451, w450) -> (resulting string=w433:string)  [unwired: 2 in, 1 out]
                        n224 = case shown="True" w432 {
                          tunnel: [T4."replace or create with confirmation" ("operation (0:open)") T4."replace or create" ("operation (0:open)")] -> w431
                          frame False {
                          }
                          frame True {
                          }
                        }
                        n225 = Concatenate Strings(w449, "\\\\" ("string"), w445, "_", "par", ".", w442) -> (w441:string)
                        n226 = String To Path(string=w441) -> (path=w435:path)
                        n227 = Open/Create/Replace File(file path (use dialog)=w435, operation (0:open)=w431, access (0:read/write)=enum16{"read/write", "read-only", "write-only"}."write-only") -> (refnum out=w437:refnum<file>, error out=w440:errorcluster)  [unwired: 3 in, 1 out]
                        n228 = Write to Text File(file (use dialog)=w437, text=w433, error in=w440) -> (refnum out=w438:refnum<file>, error out=w439:errorcluster)  [unwired: 1 in, 1 out]
                        n229 = Close File(refnum=w438, error in=w439) -> (error out=w436:errorcluster)  [unwired: 1 out]
                        n230 = call <vilib>:"Simple Error Handler.vi"("error in (no error)"=w436) -> ()  [unwired: 4 in, 5 out]
                      }
                    }
                    n231 = local write "Stop"(FALSE ("Stop")) -> ()
                  }
                }
              }
            }
          }
        }
        n232 = Wait (ms)(milliseconds to wait=u32 100) -> ()  [unwired: 1 out]
      }
    }
    frame #2 {
      n233 = Current VI's Path() -> (path=w472:path)
      n234 = Strip Path(path=w472) -> (stripped path=w473:path)  [unwired: 1 out]
      n235 = Build Path(base path=w473, name or relative path="Data_get.cfg") -> (appended path=w475:path)
      n236 = call "SaveControlValues.vi"("file path"=w475, "vi path"=w472) -> ("error out"=w474:errorcluster)
      n237 = call <vilib>:"Simple Error Handler.vi"("error in (no error)"=w474) -> ()  [unwired: 4 in, 5 out]
    }
  }
